vi "Exit Check.vi"(8 "error in (no error)":errorcluster) -> (0 "error out":errorcluster, 1 "Exit?":bool)   [LabVIEW 2018]
uses:
  Exit.lvlib
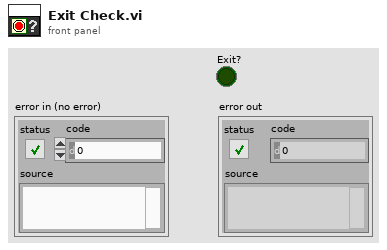
[diagram p1: front panel]
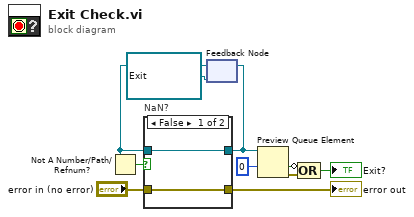
[diagram p0: block diagram]
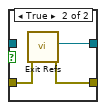
[diagram p2: hidden frame]
diagram:
  n1 = feedback #1(refnum<queue> refnum ("Exit SEQ")) -> (w10:refnum<queue>)
  n2 = Not A Number/Path/Refnum?(number/path/refnum=w10) -> (NaN/Path/Refnum?=w9:bool)
  n3 = case "NaN?" shown="False" w9 {
    tunnel: w10 -> [w12 _]
    tunnel: [w12 w15] -> w5
    tunnel: "error in (no error)" -> [w11 w14]
    tunnel: [w11 w13] -> w7
    frame False {
    }
    frame True {
      n4 = call "Exit Refs.vi"("error in (no error)"=w14) -> ("error out"=w13:errorcluster, "Exit SEQ"=w15:refnum<queue>)  [unwired: 7 in, 2 out]
    }
  }
  "error out" <- w7
  n5 = feedback-in #1(w5) -> ()
  n6 = Preview Queue Element(queue=w5, timeout in ms (-1)=0) -> (timed out?=w2:bool, error out=w3:errorcluster)  [unwired: 1 in, 2 out]
  n7 = Compound Arithmetic op=OR(invert w2, w3) -> (→"Exit?":bool)
